vi "Write TimeStampSampledInReplay.vi"(8 "error in (no error)":errorcluster, 10 "TimeStampSampledInReplay":string, 11 "Game in":refnum<class "Game.lvclass">) -> (0 "error out":errorcluster, 3 "Game out":refnum<class "Game.lvclass">)   [LabVIEW 2020, in "Game.lvclass"]
uses:
  Game.lvclass
  Game.lvclass/Game.ctl
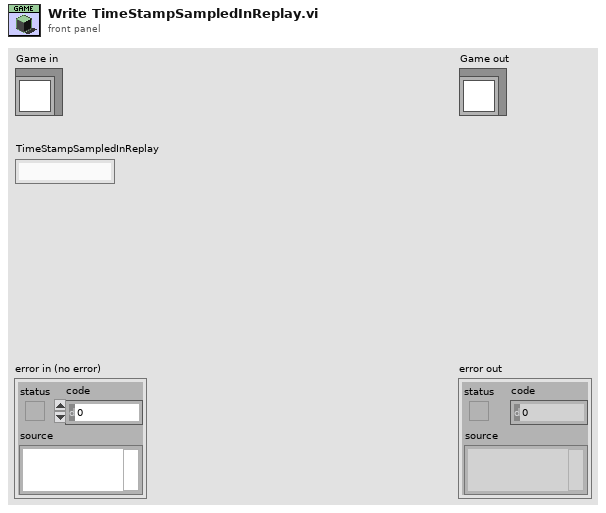
[diagram p1: front panel]
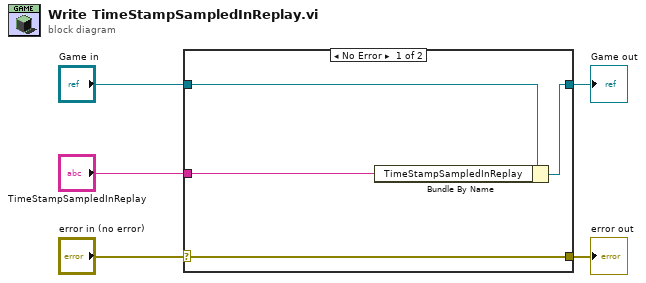
[diagram p0: block diagram]
diagram:
  n1 = case shown="No Error" "error in (no error)" {
    selector: "error in (no error)" -> [w9 w10]
    tunnel: [w9 w10] -> w4
    tunnel: [w7 w11] -> w2
    tunnel: "Game in" -> [w8 w11]
    tunnel: "TimeStampSampledInReplay" -> [w6 _]
    frame No Error {
      n2 = Bundle By Name(cluster=w8, "TimeStampSampledInReplay"=w6) -> (w7:refnum<class "Game.lvclass">)
    }
    frame Error {
    }
  }
  "error out" <- w4
  "Game out" <- w2
